vi "Read Formatters.vi"(8 "error in (no error)":errorcluster, 11 "OnTheFlyReport Config in":refnum<class "OnTheFlyReport Config.lvclass">) -> (0 "error out":errorcluster, 2 "Formatters":refnum<class "Formatter Config.lvclass">[](array[class]), 3 "OnTheFlyReport Config out":refnum<class "OnTheFlyReport Config.lvclass">)   [LabVIEW 2015, in "OnTheFlyReport Config.lvclass"]
uses:
  OnTheFlyReport Config.lvclass
  Report Formatters/Base Class/Config/Formatter Config.lvclass
  OnTheFlyReport Config.lvclass/OnTheFlyReport Config.ctl
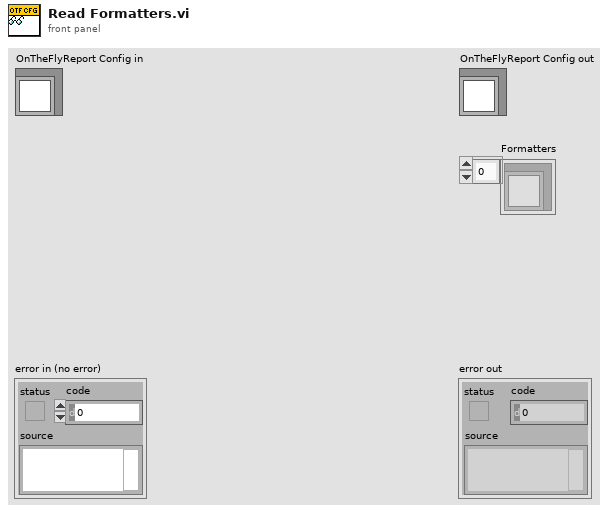
[diagram p1: front panel]
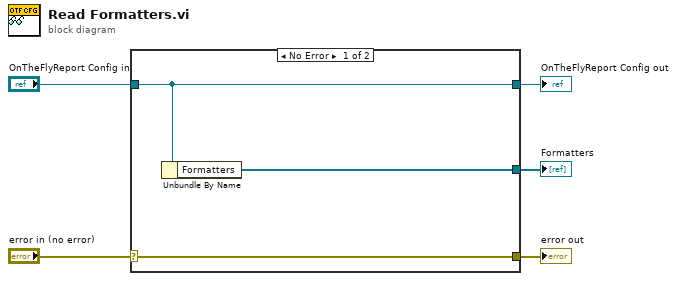
[diagram p0: block diagram]
diagram:
  n1 = case shown="No Error" "error in (no error)" {
    selector: "error in (no error)" -> [w8 w9]
    tunnel: [w8 w9] -> w4
    tunnel: [w7 w10] -> w2
    tunnel: "OnTheFlyReport Config in" -> [w7 w10]
    tunnel: [w6 _] -> w1
    frame No Error {
      n2 = Unbundle By Name(w7) -> ("Formatters"=w6:refnum<class "Formatter Config.lvclass">[])
    }
    frame Error {
    }
  }
  "error out" <- w4
  "OnTheFlyReport Config out" <- w2
  "Formatters" <- w1
